vi "sum.vi"(6 "Numeric 2":dbl, 7 "Numeric":dbl) -> (0 "B":bool[](array[boolean]), 1 "A+B 2":bool[][](array[boolean]), 2 "A":bool[](array[boolean]), 3 "A+B":dbl)   [LabVIEW 2020]
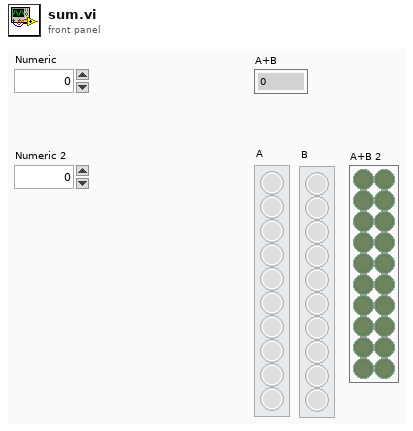
[diagram p1: front panel]
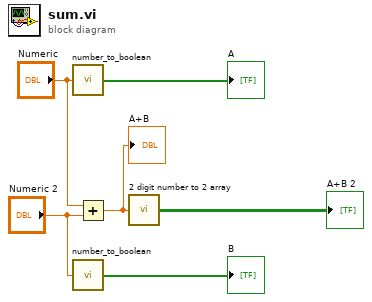
[diagram p0: block diagram]
diagram:
  n1 = call "number_to_boolean.vi"("A in"="Numeric") -> ("A out"=→"A":bool[])
  n2 = call "number_to_boolean.vi"("A in"="Numeric 2") -> ("A out"=→"B":bool[])
  n3 = Add(x="Numeric", y="Numeric 2") -> (x+y=w5:dbl)
  "A+B" <- w5
  n4 = call "2 digit number to 2 array.vi"("Numeric"=w5) -> ("transposed array"=→"A+B 2":bool[][])
